vi "Settings_DeleteEmptyCases.vi"(4 "ItemNames":string[][](array[string])) -> (1 "ItemNames w/ empty cases deleted":string[][](array[string]))   [LabVIEW 2020]
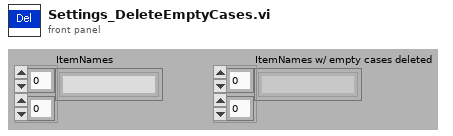
[diagram p1: front panel]
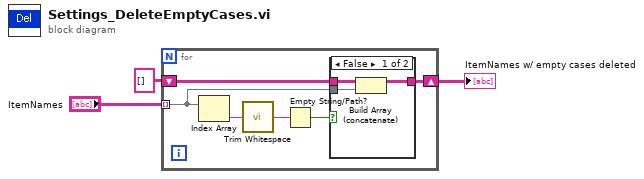
[diagram p0: block diagram]
diagram:
  n1 = for {
    tunnel: "ItemNames" -> [w4] mode=indexing
    shift-right: [w5] -> w3
    shift-left: string[][] [] ("array w/ subset deleted") -> [w6]
    n2 = Index Array(array=w4) -> (element=w9:string)  [unwired: 1 in]
    n3 = call <vilib>:"Trim Whitespace.vi"("string"=w9) -> ("trimmed string"=w8:string)  [unwired: 1 in]
    n4 = Empty String/Path?(string/path=w8) -> (empty?=w7:bool)
    n5 = case shown="False" w7 {
      tunnel: w6 -> [w12 w13]
      tunnel: [w10 w13] -> w5
      tunnel: w4 -> [w11 _]
      frame False {
        n6 = Build Array (concatenate)(w12, w11) -> (w10:string[][])
      }
      frame True {
      }
    }
  }
  "ItemNames w/ empty cases deleted" <- w3
